vi "count rate.vi"() -> ()   [LabVIEW 2014]
uses:
  <vilib>/Platform/TimedLoop/XDataNode/timing_clust.ctl
  <vilib>/Platform/TimedLoop/XDataNode/nitl_modes.ctl
  <vilib>/Platform/TimedLoop/XDataNode/wakeup.ctl
  <vilib>/imath/engines/lvmath2/RunTimeEngine/RangeToken/NIMS_Range.vi
  <instcachedir>/0/NIMS_Range_9BCE657718DF4976A877346C61F22738.lvgen/NIMS_Range_9BCE657718DF4976A877346C61F22738_003.vi
  <vilib>/imathl/engines/lvmath/Functions/Error Handling/Create Error.vi
  <vilib>/imath/engines/lvmath2/RunTimeEngine/NodeEndStatement/NIMS_NodeEndStatement_Output.vi
  <instcachedir>/0/NIMS_NodeEndStatement_Output_53EC0D466D134D7ABD903AC30B43404B.lvgen/NIMS_NodeEndStatement_Output_53EC0D466D134D7ABD903AC30B43404B_014.vi
  <vilib>/imath/engines/lvmath2/RunTimeEngine/ErrorHandling/NIMS_Finalize Error.vi
  <vilib>/Utility/file.llb/Write To Spreadsheet File (I64).vi
  <vilib>/platform/TimedLoop/XDataNode/XDataNode.xnode
  <vilib>/Platform/TimedLoop/XDataNode/XDNodeRunTimeDep.lvlib
panel:
  in  "Aquisition Time (s)":i64
  in  "Period (s)":i64=1000
  out "Waveform Graph":i32[](graph)
  out "Array":i32[](array[numeric])
  out "counts per second":dbl(knob) scale=0.0..100.0
  in  "stop":bool
  # "Demo count rate VI for Physics 434"
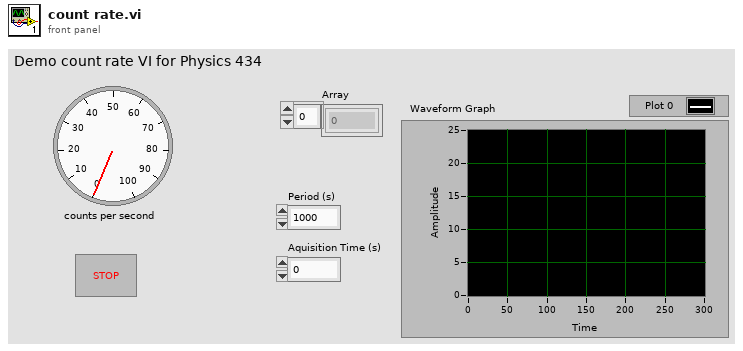
[diagram p1: front panel]
types:
  T1 = typedef "XDNodeRunTimeDep.lvlib/timing_clust.ctl" = cluster{"Expected End [f-1]":u64, "Actual End [f-1]":u64, "Finished Late? [f-1]":bool, "Expected End [i-1]":u64, "Actual End [i-1]":u64, "Finished Late? [i-1]":bool, "Expected Start [i]":u64, "Actual Start [i]":u64, "Expected Start [f]":u64, "Actual Start [f]":u64, "Source Name":string, "Structure Name":string, "Period":i64, "Deadline":i64, "Offset":i64, "Start":i64, "Priority":i32, "Timeout":i32, "Mode":T2, "Wakeup Reason":T3, "Error":errorcluster, "Source Type":string, "Secondary Source Type":string, "Global End Time":u64, "Global Start Time":u64, "Frame Duration":u64, "Iteration Duration":u64, "Assigned CPU":i32, "I/O Scan Engine Mode":u32}
  T2 = typedef "XDNodeRunTimeDep.lvlib/nitl_modes.ctl" = enum32{"No Change", "Process missed periods, maintain original phase", "Discard missed periods, maintain original phase", "Process missed periods, ignore original phase", "Discard missed periods, ignore original phase"}
  T3 = typedef "XDNodeRunTimeDep.lvlib/wakeup.ctl" = enum32{"Normal", "Aborted", "Asynchronous wakeup", "Timing source error", "Timed loop error", "Timeout"}
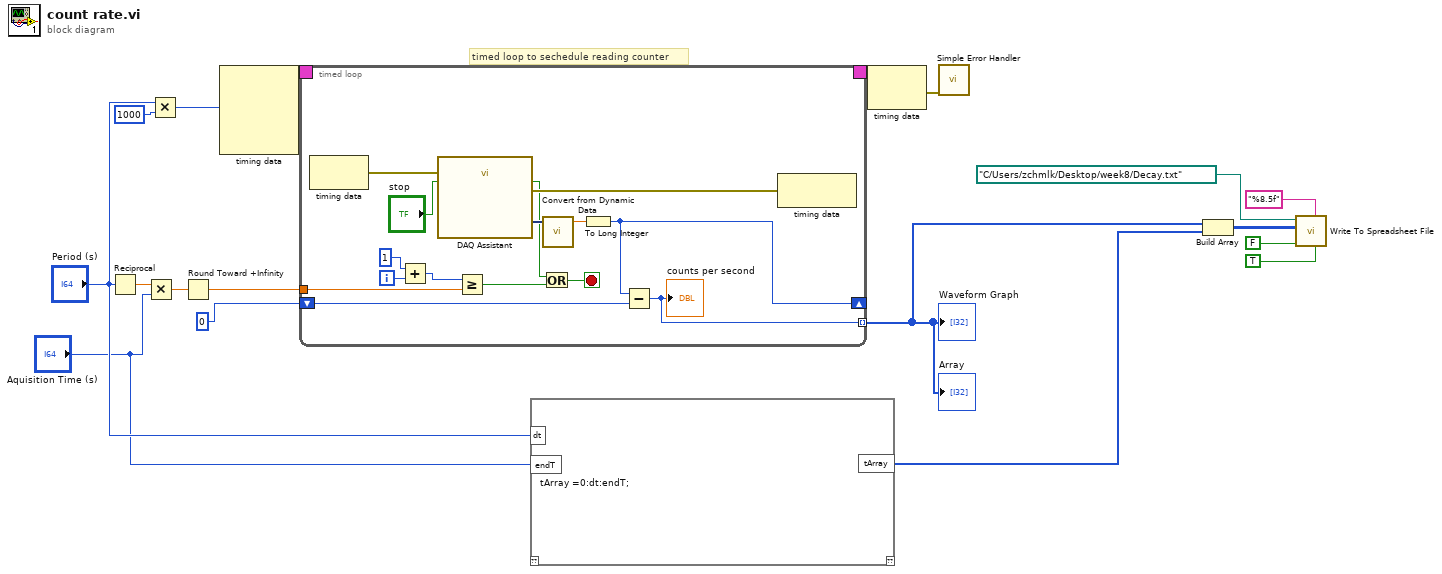
[diagram p0: block diagram]
diagram:
  # "timed loop to sechedule reading counter"
  n1 = Reciprocal(x="Period (s)") -> (1/x=w13:dbl)
  n2 = Multiply(x=w13, y="Aquisition Time (s)") -> (x*y=w12:dbl)
  n3 = Multiply(x="Period (s)", y=1000) -> (x*y=w11:i64)
  n4 = Round Toward +Infinity(x=w12) -> (ceil(x): smallest int >= x=w4:dbl)
  n5 = node-c288(w11) -> (w18:T1)  [unwired: 3 in]
  n6 = timed-loop {
    timing: w18 -> [_]
    timing-out: [_] -> w17
    shift-right: [w30] -> _
    shift-left: 0 -> [w32]
    tunnel: [w26] -> w5 mode=indexing
    tunnel: w4 -> [w22]
    i -> [w25]
    stop <- w21 stop-if-true
    n7 = node-c288() -> (w27:errorcluster)  [unwired: 1 in]
    n8 = Add(x=1, y=w25) -> (x+y=w23:i32)
    n9 = call "DAQ Assistant"("error in"=w27, "stop (F)"="stop") -> ("data"=w33:dynamicdata, "stopped"=w20:bool, "error out"=w28:errorcluster)  [unwired: 14 in, 1 out]
    n10 = Greater Or Equal?(x=w23, y=w22) -> (x >= y?=w19:bool)
    n11 = Or(x=w20, y=w19) -> (x .or. y?=w21:bool)
    n12 = call "Convert from Dynamic Data"("Dynamic Data Type"=w33) -> ("Scalar"=w29:dbl)  [unwired: 3 in]
    n13 = To Long Integer(number=w29) -> (32bit integer=w30:i32)
    n14 = Subtract(x=w30, y=w32) -> (x-y=w26:i32)
    "counts per second" <- w26
    n15 = node-c288(w28) -> ()  [unwired: 1 out]
  }
  "Array" <- w5
  "Waveform Graph" <- w5
  n16 = mathscript code="tArray =0:dt:endT;"("dt"="Period (s)", "endT"="Aquisition Time (s)") -> ("tArray"=w1:i64[])  [unwired: 1 in, 1 out]
  n17 = node-c288(w17) -> (w15:errorcluster)
  n18 = call <vilib>:"Simple Error Handler.vi"("error in (no error)"=w15) -> ()  [unwired: 4 in, 5 out]
  n19 = Build Array(w5, w1) -> (w7:i64[][])
  n20 = call-poly <vilib>:"Write To Spreadsheet File.vi"("transpose? (no:F)"=TRUE, "format (%d)"="%8.5f", "append to file? (new file:F)"=FALSE, "2D data"=w7, "file path (dialog if empty)"=path "C:/Users/zchmlk/Desktop/week8/Decay.txt") -> ()  [unwired: 3 in, 1 out]
